vi "zern2slopes.vi"(8 "error in (no error)":errorcluster, 9 "Zern coef in":sgl[](array[numeric]), 10 "Zern index in":i32[](array[numeric]), 11 "HasoSlopes in":refnum<class "HasoSlopes.lvclass">) -> (0 "error out":errorcluster, 1 "Zern pupil out":refnum<class "Pupil.lvclass">, 2 "ModalCoef out":refnum<class "ModalCoef.lvclass">, 3 "HasoSlopes out":refnum<class "HasoSlopes.lvclass">)   [LabVIEW 2018]
uses:
  <userlib>/WaveKit.lib/Controls/HasoSlopes.lvclass
  <userlib>/WaveKit.lib/Classes/ModalCoef/ModalCoef.lvclass
  <userlib>/WaveKit.lib/Controls/Pupil.lvclass
  <userlib>/WaveKit.lib/Controls/WavefrontModalReconstructionType.ctl
  <userlib>/WaveKit.lib/Controls/ZernikeModalPrefs.ctl
  <userlib>/WaveKit.lib/Controls/ZernikeProjectionPupilSetup.ctl
  <userlib>/WaveKit.lib/Controls/Point2Df.ctl
  <userlib>/WaveKit.lib/Controls/CircularPupilDetectionParams.ctl
  <userlib>/WaveKit.lib/Controls/PupilDetectionOption.ctl
  <userlib>/WaveKit.lib/Controls/CircularAutoDetectionOptions.ctl
  <userlib>/WaveKit.lib/Controls/PupilDetectionMode.ctl
  <userlib>/WaveKit.lib/Classes/ComputePhaseSet/ComputePhaseSet.lvclass
  <userlib>/WaveKit.lib/Controls/WavefrontReconstructionMode.ctl
  <vilib>/Analysis/1siggen.llb/Ramp Pattern by Delta.vi
  <vilib>/Analysis/NI_AALBase.lvlib
panel:
  # "Zern index in: 1D array, no more than 32 elements, each element value 1~32\nZern coef in: 1D array, coefficients corresponding to the indexes in Zern index in"
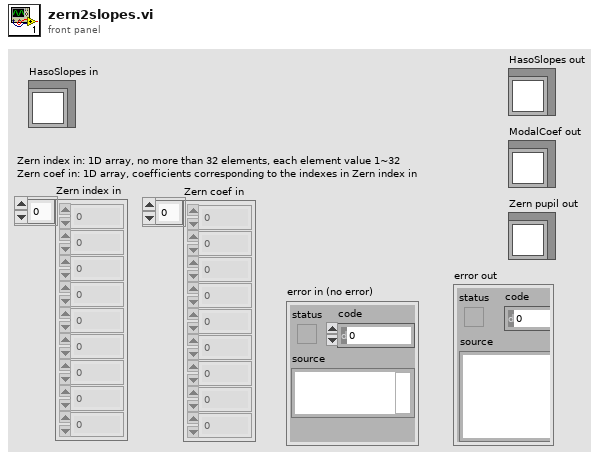
[diagram p1: front panel]
types:
  T1 = typedef "WavefrontReconstructionMode.ctl" = enum16{"None", "Modal_Legendre", "Modal_Zernike", "Zonal", "Modal_Zonal_Zernike", "Modal_Zonal_Legendre"}
  T2 = typedef "CircularPupilDetectionParams.ctl" = cluster{"PupilDetectionOption":T3, "AutoDetectionOption":T4, "PupilDetectionMode":T5, "CentralOccultationDetection":bool}
  T3 = typedef "PupilDetectionOption.ctl" = enum16{"Manual", "Automatic"}
  T4 = typedef "CircularAutoDetectionOptions.ctl" = enum16{"manual_radius_auto_center", "manual_center_auto_radius", "auto_radius_auto_center"}
  T5 = typedef "PupilDetectionMode.ctl" = enum16{"inscribed", "circumscribed"}
  T6 = typedef "ZernikeModalPrefs.ctl" = cluster{"Number of coefficients":u32, "Filtered coefficients":u32[], "RMS Zernike normalization":bool, "CircularProjectionPupilDimensions":T7}
  T7 = typedef "ZernikeProjectionPupilSetup.ctl" = cluster{"Pupil center_sspp":T8, "Pupil radius_sspp":sgl}
  T8 = typedef "Point2Df.ctl" = cluster{"X":sgl, "Y":sgl}
  T9 = typedef "WavefrontModalReconstructionType.ctl" = enum16{"Legendre", "Zernike"}
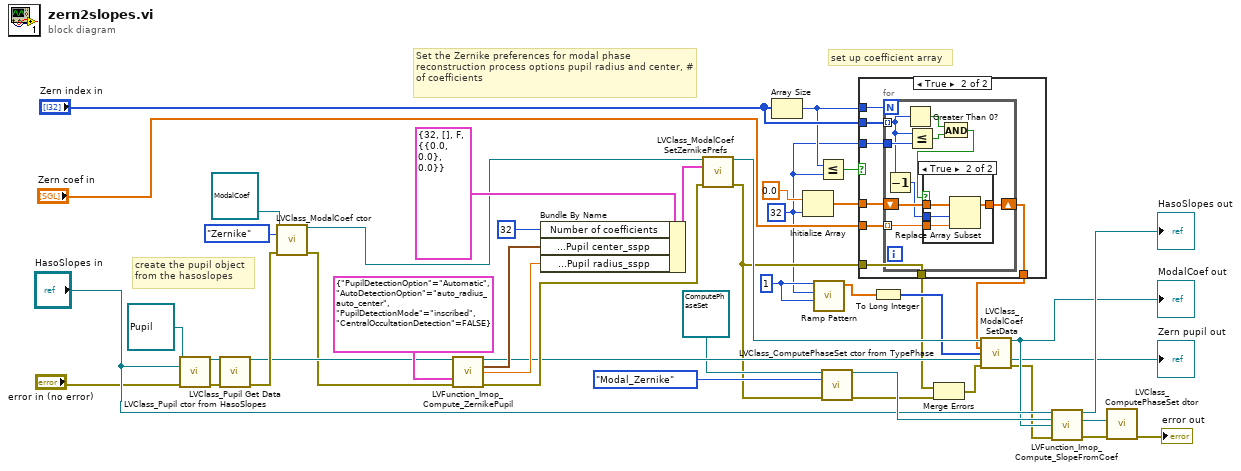
[diagram p0: block diagram]
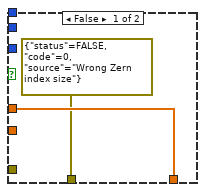
[diagram p2: hidden frame]
diagram:
  w16 = 1
  w1 = 32
  # "create the pupil object\nfrom the hasoslopes"
  # "Set the Zernike preferences for modal phase reconstruction process options pupil radius and center, # of coefficients"
  # "set up coefficient array"
  n1 = call <userlib>:"LVClass_Pupil ctor from HasoSlopes.vi"("Pupil in"=refnum<class "Pupil.lvclass"> refnum, "HasoSlopes.lvclass"="HasoSlopes in", "error in (no error)"="error in (no error)") -> ("Pupil out"=w34:refnum<class "Pupil.lvclass">, "error out"=w33:errorcluster)  [unwired: 11 in]
  n2 = call <userlib>:"LVClass_Pupil Get Data.vi"("Pupil in"=w34, "error in (no error)"=w33) -> ("Pupil out"=w31:refnum<class "Pupil.lvclass">, "error out"=w32:errorcluster)  [unwired: 11 in, 1 out]
  n3 = call <userlib>:"LVClass_ModalCoef ctor.vi"("ModalCoef in"=refnum<class "ModalCoef.lvclass"> refnum, "TypePhase"=WavefrontModalReconstructionType."Zernike", "error in (no error)"=w32) -> ("ModalCoef out"=w40:refnum<class "ModalCoef.lvclass">, "error out"=w30:errorcluster)  [unwired: 11 in]
  n4 = call <userlib>:"LVFunction_Imop_Compute_ZernikePupil.vi"("Pupil.lvclass"=w31, "CircularPupilDetectionParams"=T2 {"PupilDetectionOption"=enum."Automatic", "AutoDetectionOption"=enum."auto_radius_auto_center", "PupilDetectionMode"=enum."inscribed", "CentralOccultationDetection"=FALSE}, "error in"=w30) -> ("Pupil.lvclass"=w28:refnum<class "Pupil.lvclass">, "center"=w36:T8, "radius"=w37:sgl, "error out"=w29:errorcluster)  [unwired: 9 in]
  n5 = Bundle By Name(cluster=T6 {"Number of coefficients"=32, "Filtered coefficients"=[], "RMS Zernike normalization"=FALSE, "CircularProjectionPupilDimensions"={"Pupil center_sspp"={"X"=0.0, "Y"=0.0}, "Pupil radius_sspp"=0.0}} ("ZernikeModalPrefs"), "Number of coefficients"=u32 32, "CircularProjectionPupilDimensions.Pupil center_sspp"=w36, "CircularProjectionPupilDimensions.Pupil radius_sspp"=w37) -> (w42:T6)
  n6 = call <userlib>:"LVClass_ModalCoef SetZernikePrefs.vi"("ModalCoef in"=w40, "ZernikeModalPrefs"=w42, "error in (no error)"=w29) -> ("ModalCoef out"=w27:refnum<class "ModalCoef.lvclass">, "error out"=w2:errorcluster)  [unwired: 11 in]
  n7 = Array Size(array="Zern index in") -> (size(s)=w6:i32)
  n8 = Initialize Array(0.0, w1) -> (w13:dbl[])
  n9 = call-poly <vilib>:"Ramp Pattern.vi"("start"=w16, "end"=w1, "delta"=w16) -> ("Ramp Pattern"=w15:dbl[])  [unwired: 6 in, 2 out]
  n10 = Less Or Equal?(x=w6, y=w1) -> (x <= y?=w7:bool)
  n11 = call <userlib>:"LVClass_ComputePhaseSet ctor from TypePhase.vi"("ComputePhaseSet in"=refnum<class "ComputePhaseSet.lvclass"> refnum, "TypePhase"=WavefrontReconstructionMode."Modal_Zernike", "error in (no error)"=w2) -> ("ComputePhaseSet out"=w24:refnum<class "ComputePhaseSet.lvclass">, "error out"=w3:errorcluster)  [unwired: 11 in]
  n12 = case shown="True" w7 {
    tunnel: w6 -> [_ w54]
    tunnel: w13 -> [w47 w53]
    tunnel: [w47 w52] -> w12
    tunnel: "Zern index in" -> [_ w51]
    tunnel: "Zern coef in" -> [_ w50]
    tunnel: [errorcluster {"status"=FALSE, "code"=0, "source"="Wrong Zern index size"} ("error out") w49] -> w4
    tunnel: w2 -> [_ w49]
    tunnel: w1 -> [_ w48]
    frame False {
    }
    frame True {
      n13 = for {
        N: w54 -> [_]
        shift-right: [w62] -> w52
        shift-left: w53 -> [w63]
        tunnel: w51 -> [w58] mode=indexing
        tunnel: w50 -> [w61] mode=indexing
        tunnel: w48 -> [w59]
        n14 = Decrement(x=w58) -> (x-1=w60:i32)
        n15 = Greater Than 0?(x=w58) -> (x > 0?=w57:bool)
        n16 = Less Or Equal?(x=w58, y=w59) -> (x <= y?=w56:bool)
        n17 = And(x=w57, y=w56) -> (x .and. y?=w55:bool)
        n18 = case shown="True" w55 {
          tunnel: w60 -> [_ w68]
          tunnel: w63 -> [w64 w67]
          tunnel: [w64 w66] -> w62
          tunnel: w61 -> [_ w65]
          frame False {
          }
          frame True {
            n19 = Replace Array Subset(array=w67, new element=w65, index=w68) -> (w66:dbl[])
          }
        }
      }
    }
  }
  n20 = To Long Integer(number=w15) -> (32bit integer=w14:i32[])
  n21 = Merge Errors(w4, w3) -> (w5:errorcluster)
  n22 = call <userlib>:"LVClass_ModalCoef SetData.vi"("ModalCoef in"=w27, "coef"=w12, "index"=w14, "Pupil.lvclass"=w28, "error in (no error)"=w5) -> ("ModalCoef out"=w18:refnum<class "ModalCoef.lvclass">, "Pupil (dup)"=→"Zern pupil out":refnum<class "Pupil.lvclass">, "error out"=w17:errorcluster)  [unwired: 7 in, 1 out]
  "ModalCoef out" <- w18
  n23 = call <userlib>:"LVFunction_Imop_Compute_SlopeFromCoef.vi"("HasoSlopes.lvclass"="HasoSlopes in", "ComputePhaseSet"=w24, "ModalCoef.lvclass"=w18, "error IO"=w17) -> ("HasoSlopes.lvclass"=→"HasoSlopes out":refnum<class "HasoSlopes.lvclass">, "ComputePhaseSet (dup)"=w23:refnum<class "ComputePhaseSet.lvclass">, "error IO out"=w20:errorcluster)  [unwired: 8 in, 1 out]
  n24 = call <userlib>:"LVClass_ComputePhaseSet dtor.vi"("ComputePhaseSet in"=w23, "error in (no error)"=w20) -> ("error out"=→"error out":errorcluster)  [unwired: 12 in, 1 out]
